vi "PH_BeamlineController.get Boolean Status Attributes.vi"(0 "VI in":refnum<vi>, 2 "Name":string, 5 "error in (no error)":errorcluster) -> (14 "VI out":refnum<vi>, 15 "Status Tags":cluster{"Name":string, "Status":T1}[](array[cluster]) {"Status" items=["no info", "off/false/out", "on/true/in", "Failure", "Alarm", "Status 1", "Status 2", "Status 3"]}, 16 "Status":T1 items=["no info", "off/false/out", "on/true/in", "Failure", "Alarm", "Status 1", "Status 2", "Status 3"], 17 "index of element":i32, 18 "Tag":cluster{"Name":string, "Status":T1} {"Status" items=["no info", "off/false/out", "on/true/in", "Failure", "Alarm", "Status 1", "Status 2", "Status 3"]}, 19 "error out":errorcluster)   [LabVIEW 2014, in "PH_BeamlineController.lvlib"]
uses:
  PH_BeamlineController.lvlib
  PH_Basics/PH_StatusHandler/PH_StatusHandler.Status.ctl
  PH_Basics/PH_StatusHandler/PH_StatusHandler.lvlib
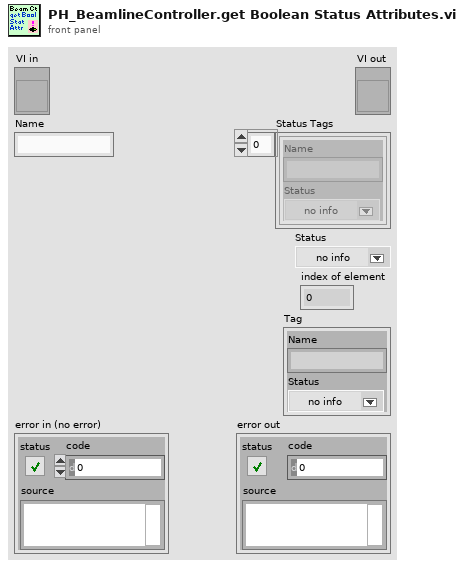
[diagram p1: front panel]
types:
  T1 = typedef "PH_StatusHandler.lvlib/PH_StatusHandler.Status.ctl" = i16
  T2 = typedef "PH_BeamlineController.lvlib/PH_BeamlineController.i attribute.ctl" = cluster{"Vacuum Exp LB":cluster{"Channel":string, "Limit [mbar]":dbl, "Pressure [mbar]":dbl, "GUI Ref":refnum<vi>}, "Sources":T3[], "PA DP Targets":T5[], "Path":cluster{"Source":T4, "PA DP Target":T6, "Target":T7}, "Targets":cluster{"Name":T7, "GUI Ref":refnum<vi>, "Current State":bool, "Wanted State":bool, "Enabled":bool}[], "Status Tags":cluster{"Name":string, "Status":T1}[], "special GUI Refs":T8}
  T3 = typedef "PH_BeamlineController.lvlib/PH_BeamlineController.Source Attributes.ctl" = cluster{"Name":T4, "GUI Ref":refnum<vi>, "Current State":bool, "Wanted State":bool}
  T4 = typedef "PH_BeamlineController.lvlib/PH_BeamlineController.Sources.ctl" = enum16{"None", "YLF", "fs-Frontend", "ns-Frontend", "YLF and ns-Frontend", "fs- and ns-Frontend"}
  T5 = typedef "PH_BeamlineController.lvlib/PH_BeamlineController.PA DP Target Attributes.ctl" = cluster{"Name":T6, "GUI Ref":refnum<vi>, "Current State":bool, "Wanted State":bool, "Enabled":bool}
  T6 = typedef "PH_BeamlineController.lvlib/PH_BeamlineController.PA DP Targets.ctl" = enum16{"None", "Dump PA Delayed Beam", "Dump PA Undelayed Beam", "Dumps PA Delayed and Undelayed Beam"}
  T7 = typedef "PH_BeamlineController.lvlib/PH_BeamlineController.Targets.ctl" = enum16{"None", "PreAmp", "Dump Exp Laserlab", "Exp Laserlab", "Calorimeter", "Dump Exp Laserbay", "Exp Laserbay", "Dump Exp Z6", "Exp Z6"}
  T8 = typedef "PH_BeamlineController.lvlib/PH_BeamlineController.special GUI Refs.ctl" = cluster{"PA-Backreflection-Meas":refnum<vi>, "fs_Synchrolock_Watch":refnum<vi>}
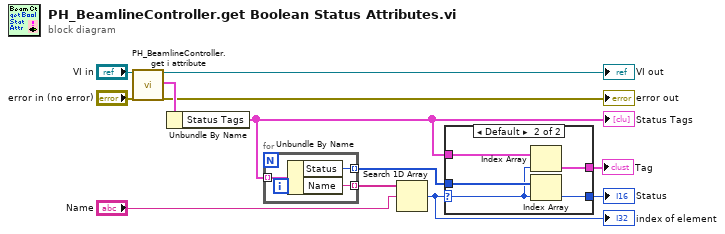
[diagram p0: block diagram]
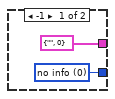
[diagram p2: hidden frame]
diagram:
  n1 = call "PH_BeamlineController.get i attribute.vi"("i ref in"="VI in", "error in (no error)"="error in (no error)") -> ("i ref out"=→"VI out":refnum<vi>, "i attribute"=w8:T2, "error out"=→"error out":errorcluster)  [unwired: 15 in]
  n2 = Unbundle By Name(w8) -> ("Status Tags"=w2:cluster{"Name":string, "Status":T1}[])
  "Status Tags" <- w2
  n3 = for {
    tunnel: w2 -> [w15] mode=indexing
    tunnel: [w14] -> w9 mode=indexing
    tunnel: [w13] -> w11 mode=indexing
    n4 = Unbundle By Name(w15) -> ("Status"=w13:T1, "Name"=w14:string)
  }
  n5 = Search 1D Array(1D array=w9, element="Name") -> (index of element=w3:i32)  [unwired: 1 in]
  "index of element" <- w3
  n6 = case shown="Default" w3 {
    selector: w3 -> [_ w18]
    tunnel: [w17 w22] -> w12
    tunnel: w11 -> [_ w21]
    tunnel: w2 -> [_ w20]
    tunnel: [cluster{"Name":string, "Status":T1} {"Name"="", "Status"=0} ("Tag") w19] -> w1
    frame -1 {
      w17 = T1 0 items=["no info", "off/false/out", "on/true/in", "Failure", "Alarm", "Status 1", "Status 2", "Status 3"] ("Status")
    }
    frame Default {
      n7 = Index Array(array=w20, index=w18) -> (element=w19:cluster{"Name":string, "Status":T1})
      n8 = Index Array(array=w21, index=w18) -> (element=w22:T1)
    }
  }
  "Status" <- w12
  "Tag" <- w1
